vi "Find Caption in 2D [ ].vi"(6 "Class ID":u32, 7 "Langues/Languages":u8, 8 "error in (no error)":errorcluster, 10 "Nom":string, 11 "Array IN":string[][](array[string])=[["Configuration Caption", "Français", "Anglais"], ["Nom de l'essai", "Nom de l'essai", "Test name"], ["Durée", "Durée", "Duration"], ["Type", "Type", ""], ["Surface", "Surface", "Area"], ["Nbre cellules", "Nombre de cellules", "Cells number"], [" T Essai affiché", "Températures visées (°C):", "Températures Set Point (°C):"], ["Bouteille eau H2", "Bouteille eau H2", "Water Bottle H2"], ["Ligne H2", "Ligne H2", "H2 Line"], ["Bouteille eau O2 ", "Bouteille eau O2 ", "Water Bottle 2"], ["Ligne O2", "Ligne O2", "O2 Line"], ["Température pile à combustible", "Température pile à combustible", "Fuel Cell Temperature"], ["% RH H2", "% RH H2", "% RH H2"], ["% RH O2", "% RH O2", "% RH O2"], [" Humidité relative", "Humidités résultantes:", "Calculated Humidity:"], [" Débit durant durant l'essai ml/min:", " Débit durant durant l'essai (ml/min):", " Flow during testi (ml/min):"], ["Ligne H2", "Ligne H2", "H2 Line"], ["Ligne O2", "Ligne O2", "O2 Line"], ["Purge", "Purge à l'azote (ml/min)", "Nitrogen Purge (ml/min)"], ["Débit (ml/min)", "LIgne N2", "N2 Line"], ["Nombres de minutes", "Temsp (min)", "Duration (min.)"], ["Variation de gaz (ml/min)", "Taux de variation de gaz (ml/min/min)", "Variation Rate (ml/min/min)"], ["Augmentation", "Augmentation", "Increase"], ["Diminution", "Diminution", "Decrease"], ["Choisir cycle activation", "Définir", "Set"], ["Valeurs max polarisation", "Valeurs des polarisations (à P max)", "Polarization Values (at P max)"], ["Mode de polarisation", "Mode de polarisation ", "Polarization Mode"], ["Attente entre les mesures (sec)", "Attente entre les mesures (sec)", "Holding Time (s)"], ["Balayage unité", "Type de balyage", "Scan Type"], ["Balayage à la fin ", "Courbe de polarisation à la fin?", "Polarization Curve at the End?"], ["Balayage au début ", "Courbe de polarisation au début?", "Polarization Curve at Start?"], ["Attendre après polarisation initiale ", "Confirmation de l'opérateur pour continuer  \naprès la polarisation initiale?", "COnfirmation by the operator after\nthe initial polarization?"], ["CE Balayage mode ", "Type de Balayage", "Scan Type"], ["Choisir durant l'essai", "Définir", "Set"], ["Voltage (V)", "Voltage (V)", "Voltage (V)"], ["Current (A)", "Courant (A)", "Current (A)"], ["Power (watts)", "Puissance (W)", "Power (watts)"], ["Resistance (W)", "Reisistance (Ohm)", "Resistance (Ohm)"], ["CE Valeurs max", "Valeurs limites", "Maximum Values"]]) -> (0 "error out":errorcluster, 2 "Légende":string, 3 "Array OUT":string[][](array[string]))   [LabVIEW 2013]
doc: "Jean-Marc Simard \nExaprom inc. 2009"
uses:
  <vilib>/Utility/error.llb/DialogType.ctl
  main.lvlib
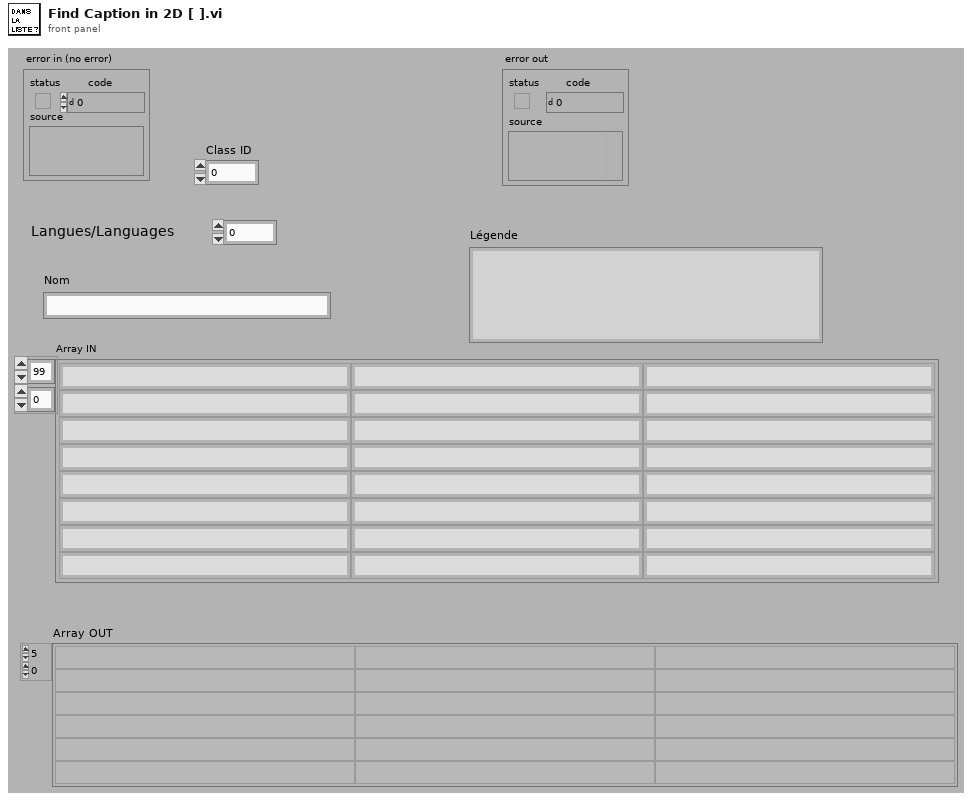
[diagram p1: front panel]
types:
  T1 = typedef "DialogType.ctl" = u16
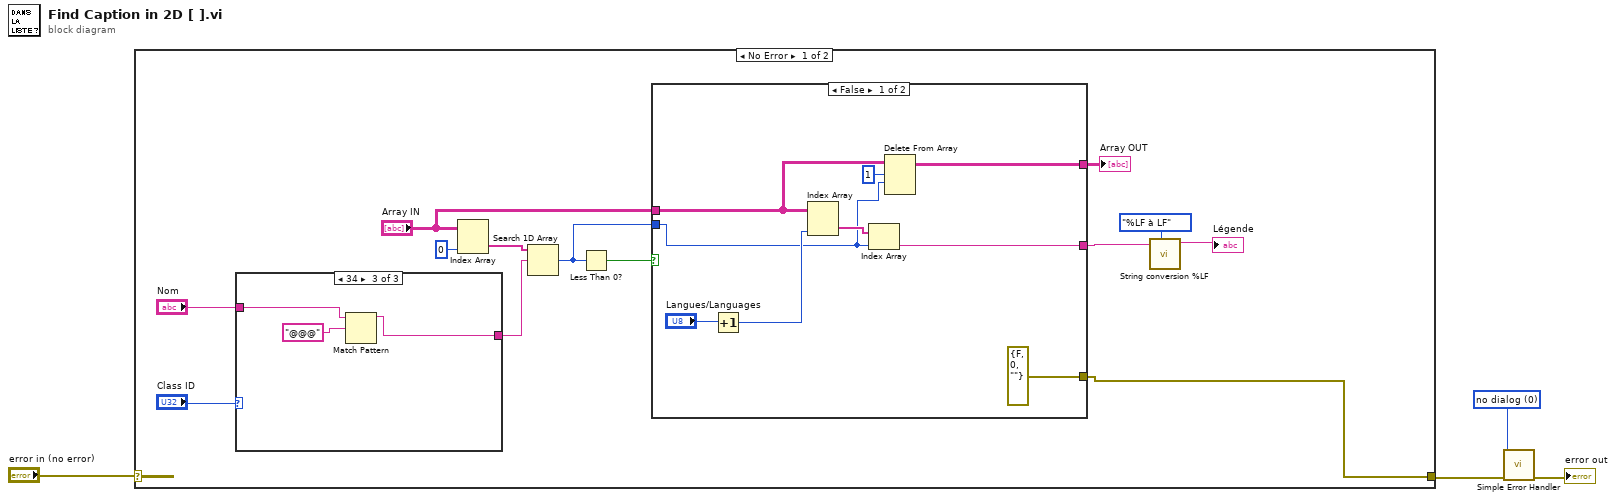
[diagram p0: block diagram]
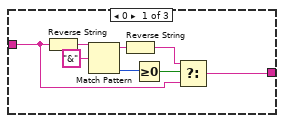
[diagram p2: hidden frame]
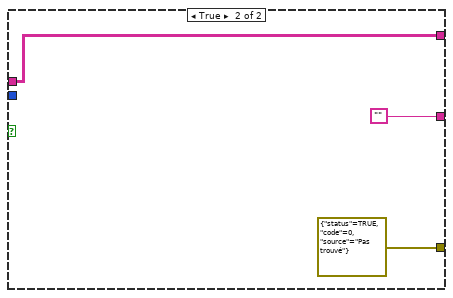
[diagram p4: hidden frame]
diagram:
  w1 = T1 0 items=["no dialog", "OK message", "continue or stop message", "OK message + warnings", "continue/stop + warnings"] ("type of dialog (OK msg:1)")
  n1 = case shown="No Error" "error in (no error)" {
    selector: "error in (no error)" -> [_ w42]
    tunnel: [w8 w42] -> w2
    frame No Error {
      n2 = case shown="34" "Class ID" {
        tunnel: "Nom" -> [w21 w26 w28]
        tunnel: [w18 w26 w27] -> w10
        frame 0 {
          n3 = Reverse String(1:w21) -> (0:w25:string)
          n4 = Match Pattern(string=w25, regular expression="&") -> (before substring=w20:string, offset past match=w23:i32)  [unwired: 3 out]
          n5 = Reverse String(1:w20) -> (0:w19:string)
          n6 = Greater Or Equal To 0?(x=w23) -> (x >= 0?=w22:bool)
          n7 = Select(t=w19, s=w22, f=w21) -> (s? t:f=w18:string)
        }
        frame 1, Default {
        }
        frame 34 {
          n8 = Match Pattern(string=w28, regular expression="@@@") -> (before substring=w27:string)  [unwired: 4 out]
        }
      }
      n9 = Index Array(array="Array IN", index (col)=0 ("disabled index (col)")) -> (element=w17:string[])  [unwired: 1 in]
      n10 = Search 1D Array(1D array=w17, element=w10) -> (index of element=w14:i32)  [unwired: 1 out]
      n11 = Less Than 0?(x=w14) -> (x < 0?=w15:bool)
      n12 = case shown="False" w15 {
        tunnel: w14 -> [w31 _]
        tunnel: "Array IN" -> [w33 w39]
        tunnel: [w35 ""] -> w6
        tunnel: [errorcluster {"status"=FALSE, "code"=0, "source"=""} ("error IO") errorcluster {"status"=TRUE, "code"=0, "source"="Pas trouvé"} ("error IO")] -> w8
        tunnel: [w30 w39] -> w12
        frame False {
          n13 = Increment(x="Langues/Languages") -> (x+1=w37:u8)
          n14 = Index Array(array=w33, index (col)=w37) -> (element=w36:string[])  [unwired: 1 in]
          n15 = Index Array(array=w36, index=w31) -> (element=w35:string)
          n16 = Delete From Array(array=w33, length=1, index (row)=w31) -> (array with subset deleted=w30:string[][])  [unwired: 1 in, 1 out]
        }
        frame True {
        }
      }
      "Array OUT" <- w12
      n17 = call "String conversion %LF.vi"("Conversion"=enum16{"LF à %LF", "%LF à LF"}."%LF à LF", "String IN"=w6) -> ("String OUT"=→"Légende":string)  [unwired: 9 out]
    }
    frame Error {
    }
  }
  n18 = call <vilib>:"Simple Error Handler.vi"("type of dialog (OK msg:1)"=w1, "error in (no error)"=w2) -> ("error out"=→"error out":errorcluster)  [unwired: 7 out]
